vi "De_Scramble.vi"(3 "rm_len":dbl[](array[numeric]), 4 "ue_index":dbl, 5 "C":dbl, 6 "demoddata":dbl[](array[numeric]), 7 "cellid":dbl, 8 "error in (no error)":errorcluster caption="错误输入（无错误）", 9 "Qm":dbl, 10 "prb_num":dbl, 11 "appended path":path) -> (0 "error IO":errorcluster, 1 "deccbc_data":dbl[][](array[numeric]))   [LabVIEW 2015]
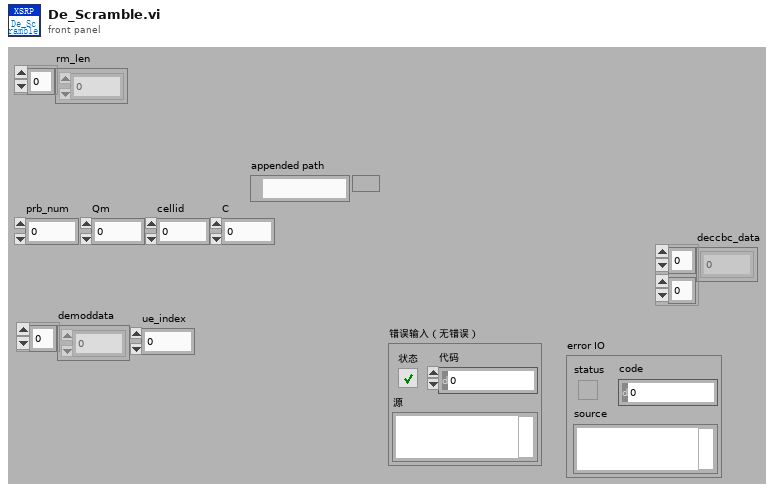
[diagram p1: front panel]
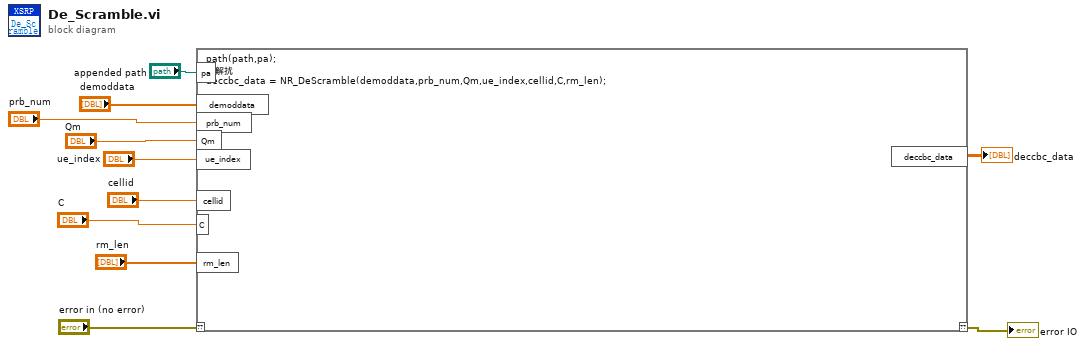
[diagram p0: block diagram]
diagram:
  n1 = script code="path(path,pa);\n%解扰\ndeccbc_data = NR_DeScramble(demoddata,prb_num,Qm,ue_index,cellid,C,rm_len);"("??"="error in (no error)", "pa"="appended path", "demoddata"="demoddata", "prb_num"="prb_num", "Qm"="Qm", "ue_index"="ue_index", "cellid"="cellid", "C"="C", "rm_len"="rm_len") -> ("??"=→"error IO":errorcluster, "deccbc_data"=→"deccbc_data":dbl[][])
